vi "Generate Item Map.vi"(8 "error in (no error)":errorcluster, 11 "Icon Decorator In":refnum<class "Icon Decorator.lvclass">) -> (0 "error out":errorcluster, 3 "Icon Decorator Out":refnum<class "Icon Decorator.lvclass">)   [LabVIEW 2020, in "Icon Decorator.lvclass"]
uses:
  Icon Decorator.lvclass
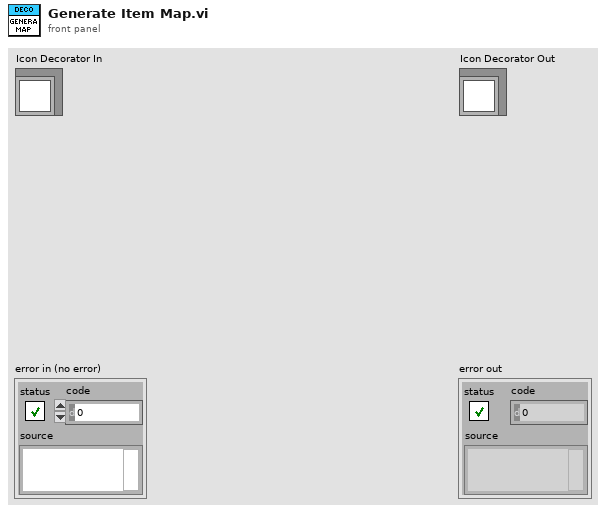
[diagram p1: front panel]
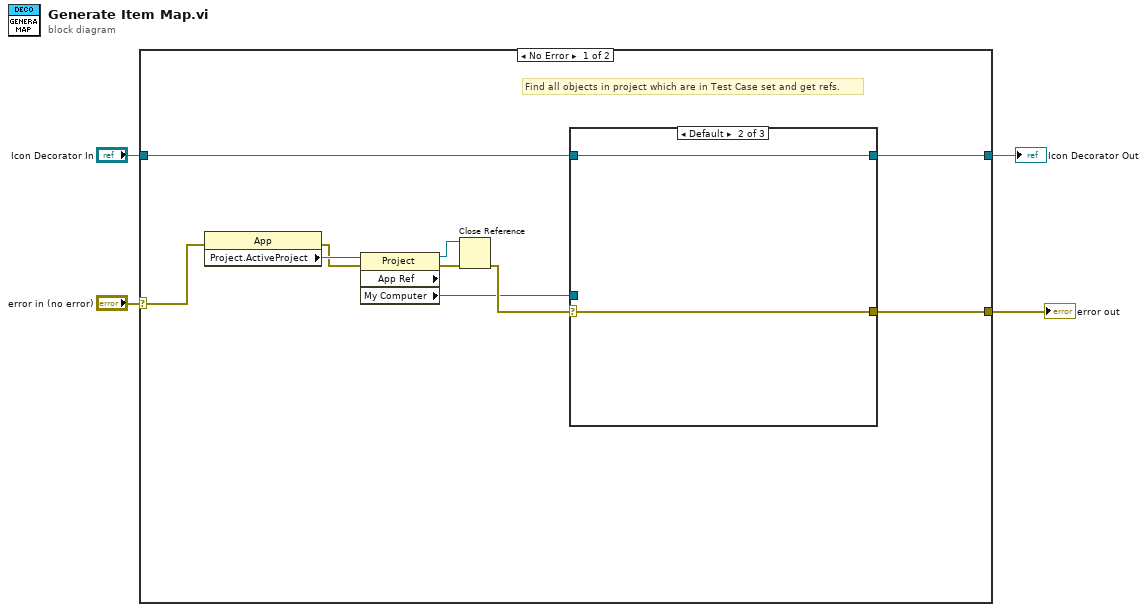
[diagram p0: block diagram]
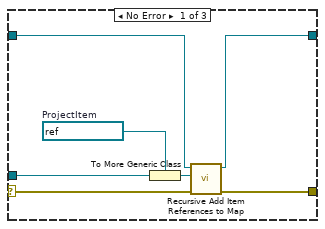
[diagram p2: hidden frame]
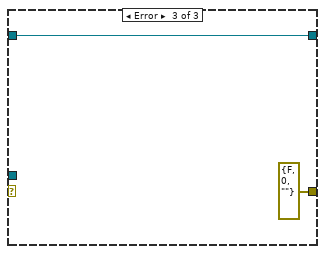
[diagram p3: hidden frame]
diagram:
  n1 = case shown="No Error" "error in (no error)" {
    selector: "error in (no error)" -> [w14 w27]
    tunnel: "Icon Decorator In" -> [w13 w26]
    tunnel: [w5 w27] -> w2
    tunnel: [w12 w26] -> w1
    frame No Error {
      # "Find all objects in project which are in Test Case set and get refs."
      n2 = property class="App"(error in=w14) -> (error out=w6:errorcluster, "Project.ActiveProject"=w9:refnum<vi>)  [unwired: 1 in, 1 out]
      n3 = property class="Project" props=["App Ref", "My Computer"](reference=w9, error in=w6) -> (reference out=w7:refnum<vi>, error out=w8:errorcluster, "My Computer"=w10:refnum<vi>)  [unwired: 1 out]
      n4 = Close Reference(reference=w7, error in (no error)=w8) -> (error out=w11:errorcluster)
      n5 = case shown="Default" w11 {
        selector: w11 -> [w17 w23 _]
        tunnel: w13 -> [w21 w22 w25]
        tunnel: [w18 w22 w25] -> w12
        tunnel: w10 -> [w16 _ _]
        tunnel: [w15 w23 errorcluster {"status"=FALSE, "code"=0, "source"=""} ("error out")] -> w5
        frame No Error {
          w19 = refnum<vi> refnum  # ProjectItem
          n6 = To More Generic Class(target class=w19, reference=w16) -> (generic class reference=w20:refnum<vi>)
          n7 = call "Recursive Add Item References to Map.vi"("error in (no error)"=w17, "ProjectItem Refnum"=w20, "Icon Decorator in"=w21) -> ("error out"=w15:errorcluster, "Icon Decorator out"=w18:refnum<class "Icon Decorator.lvclass">)  [unwired: 7 in]
        }
        frame Default {
        }
        frame Error {
        }
      }
    }
    frame Error {
    }
  }
  "error out" <- w2
  "Icon Decorator Out" <- w1
